vi "Read Data.vi"(8 "error in (no error)":errorcluster, 11 "Send Data Msg in":refnum<class "Send Data Msg.lvclass">) -> (0 "error out":errorcluster, 2 "Base Data Class.lvlib:Data":refnum<class "Data.lvclass">, 3 "Send Data Msg out":refnum<class "Send Data Msg.lvclass">)   [LabVIEW 2014, in "Send Data Msg.lvclass"]
uses:
  Send Data Msg.lvclass
  Data/Data.lvlibp/Data.lvclass
  Send Data Msg.lvclass/Send Data Msg.ctl
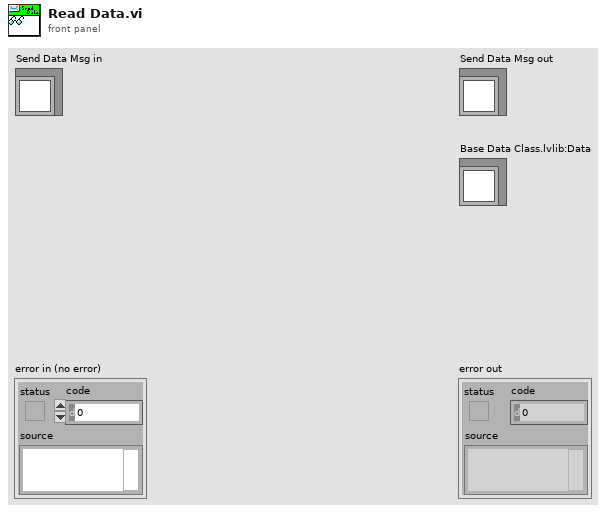
[diagram p1: front panel]
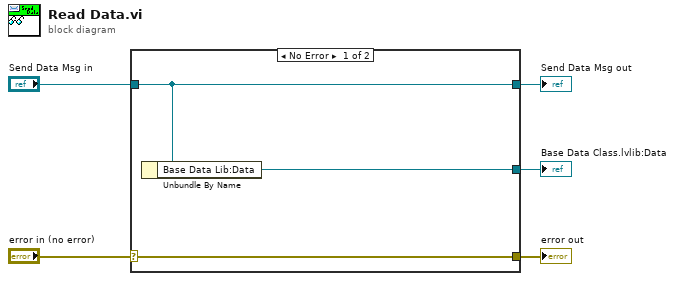
[diagram p0: block diagram]
diagram:
  n1 = case shown="No Error" "error in (no error)" {
    selector: "error in (no error)" -> [w8 w9]
    tunnel: [w8 w9] -> w4
    tunnel: [w7 w10] -> w2
    tunnel: "Send Data Msg in" -> [w7 w10]
    tunnel: [w6 _] -> w1
    frame No Error {
      n2 = Unbundle By Name(w7) -> ("Base Data Lib:Data"=w6:refnum<class "Data.lvclass">)
    }
    frame Error {
    }
  }
  "error out" <- w4
  "Send Data Msg out" <- w2
  "Base Data Class.lvlib:Data" <- w1
